vi "ClearErrors.vi"() -> ()   [LabVIEW 2014]
uses:
  <resource>/objmgr/nimcca.rc
panel:
  out "error out":errorcluster
  in  "Motion Resource":refnum<k21>="nism://SoftMotionSDI9068/Axis 1"
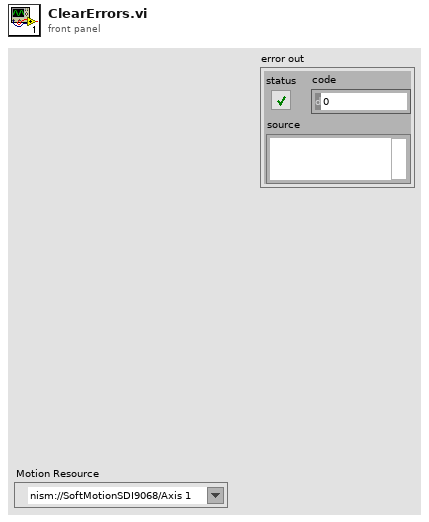
[diagram p1: front panel]
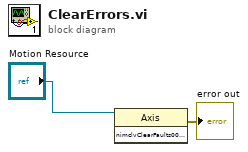
[diagram p0: block diagram]
diagram:
  n1 = invoke class="Axis" method="nimclvClearFaults00A10001"(reference="Motion Resource") -> (error out=→"error out":errorcluster)  [unwired: 2 in, 2 out]
